vi "DAC TC Temp CryoSep FP Conf.vi"(8 "error in (no error)":errorcluster, 9 "Used TC Temps":bool[](array[boolean]), 10 "Result Unit":string, 11 "Cryo Sep Results in":refnum<class "Cryo Sep Results.lvclass">) -> (0 "error out":errorcluster, 3 "Cryo Sep Results out":refnum<class "Cryo Sep Results.lvclass">)   [LabVIEW 2019, in "Results.lvlib" / "Cryo Sep Results.lvclass"]
uses:
  Cryo Sep Results.lvclass
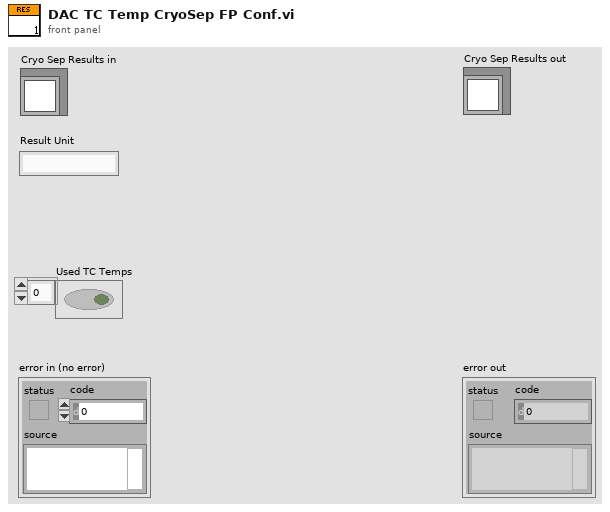
[diagram p1: front panel]
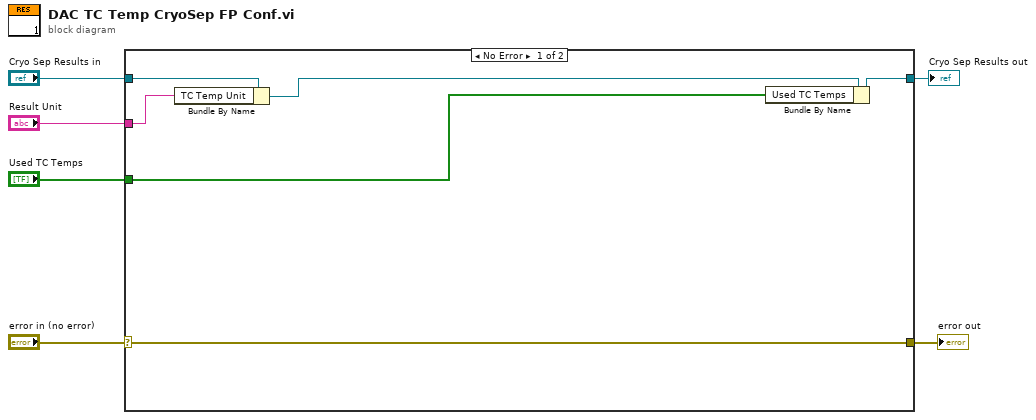
[diagram p0: block diagram]
diagram:
  n1 = case shown="No Error" "error in (no error)" {
    selector: "error in (no error)" -> [w12 w14]
    tunnel: [w12 w14] -> w5
    tunnel: [w8 w13] -> w1
    tunnel: "Cryo Sep Results in" -> [w10 w13]
    tunnel: "Result Unit" -> [w9 _]
    tunnel: "Used TC Temps" -> [w7 _]
    frame No Error {
      n2 = Bundle By Name(cluster=w10, "TC Temp Unit"=w9) -> (w11:refnum<class "Cryo Sep Results.lvclass">)
      n3 = Bundle By Name(cluster=w11, "Used TC Temps"=w7) -> (w8:refnum<class "Cryo Sep Results.lvclass">)
    }
    frame Error {
    }
  }
  "error out" <- w5
  "Cryo Sep Results out" <- w1
